vi "mfcc.vi"(1 "resoluci—n frec":dbl=21.533203125, 2 "PSD":dbl[](graph)=[3.9887404437067745e-08, 4.863361306709987e-06, 1.3039418095344414e-05, 5.070012021923156e-06, 2.6988740160259597e-08, 9.26549526636648e-08, 3.8708700843128457e-07, 5.27273770508995e-07, 1.8373351232795647e-07, 2.6971849055927445e-08, 1.1305706015574627e-07, 3.806307699408786e-08, 2.0069416323355392e-07, 2.823609797855514e-08, 5.568307171527192e-07, 4.654751624780882e-07, 1.8592522762634433e-07, 7.805098623746083e-09, 7.415656034335313e-08, 8.618601809462274e-08, 8.367973007840736e-09, 2.741395830035607e-09, 1.29708294460803e-08, 4.94468548724558e-08, 4.2508491067198684e-08, 2.5345057363752737e-09, 5.384088622693212e-09, 4.567329467519097e-10, 4.589634256892734e-08, 8.061224081254841e-08, 4.9934089467380857e-08, 4.900251155663863e-08, 6.064620630253797e-08, 1.3977491793314023e-08, 1.2377637981365425e-08, 1.2830909334877326e-08, 1.2367865096283767e-08, 2.2310979820652065e-09, 5.329299843141029e-10, 8.358860058537406e-10, 2.7965160679452414e-09, 8.57666812976728e-09, 5.0904982945537655e-09, 1.850249424215745e-08, 6.567181023968075e-09, 1.1774111924438839e-08, 2.5791701765030143e-08, 1.982423640874352e-08, 5.419962767506519e-09, 4.1419899242594406e-09, 4.689780545502817e-10, 6.653744223348867e-09, 2.6663411491893394e-08, 1.9381046099943884e-08, 3.4180900994948075e-09, 6.674963773837645e-09, 9.66181831593392e-09, 1.71947708792769e-08, 1.195261364973032e-08, 2.049897150446483e-09, 4.392273116033887e-10, 2.616427006264454e-09, 6.690001407319274e-09, 7.684978388820196e-09, 3.3903996771582425e-09, 1.2620299088279496e-09, 1.5781865769333585e-08, 6.835172346273258e-09, 4.279837116370928e-09, 1.017633364236646e-09, 1.5278934940047075e-09, 7.288208655911123e-10, 5.677716902112507e-10, 3.686854781768968e-10, 1.2948045853382716e-09, 6.441644862826187e-11, 1.7379620768753635e-09, 9.67268154903921e-08, 1.5926146703086817e-07, 1.84839387576239e-08, 1.5514964942226702e-10, 3.6806446299820845e-10, 6.391088644654868e-10, 1.2100481419233764e-09, 1.578433777229095e-09, 1.56615998978063e-09, 1.6356209328902429e-09, 7.968851827673522e-10, 1.048883110359278e-10, 3.154548207484171e-10, 6.72086666489939e-11, 5.562586170593403e-10, 1.7466042145935007e-10, 4.480068289721987e-10, 4.143358107708358e-10, 6.668260473459438e-11, 1.166302512750863e-10, 8.292201135724018e-10, 3.3781116752592635e-10, 1.388955298270216e-10, 4.1396624586413795e-10, 3.227466924577699e-10, 1.0493479042861911e-10, 1.1775778471972923e-10, 9.424146957824344e-11, 2.562400516107372e-13, 3.178514317358408e-11, 1.1402815490884768e-10, 2.593014170581146e-11, 1.0387827844257038e-10, 1.9555196850340233e-10, 9.399804236122056e-11, 1.8273331201730445e-11, 2.8943679934456845e-11, 1.2548464745442652e-10, 5.7404252467202236e-11, 3.583082697816324e-11, 1.0074456051377992e-10, 9.095619866099985e-11, 1.9214591454073945e-11, 1.7653596131622882e-11, 2.3767814754529185e-12, 2.6607109775921123e-11, 2.2175044068335442e-11, 1.1690124555337247e-11, 4.7761790450858616e-11, 4.152302479914363e-11, 5.744090546714635e-12, 6.4683935263009924e-12, 1.1770787831096862e-12, 4.5604502171813085e-12, 1.0081093160672481e-11, 2.613149358671662e-12, 1.3482181950104903e-11, 1.1131001635288938e-12, 2.5930316436774895e-11, 2.2617889198053044e-11, 3.0555023298879805e-11, 1.2999813512856096e-10, 1.1342969649559696e-10, 3.401389256701131e-11, 1.709914916053185e-11, 2.4422679377509385e-12, 1.6555985492742527e-12, 6.264935903608755e-12, 4.015636408815974e-12, 9.743669817695263e-12, 1.9242639981813654e-11, 9.976037495847763e-12, 1.065334544865495e-12, 7.606626156361599e-13, 4.924272167651513e-12, 2.7369335129743866e-12, 3.3145210049964618e-12, 8.612410770954802e-12, 3.0322149259003043e-11, 3.1739545043346e-11, 6.513310204922844e-12, 1.1414676387609523e-12, 2.531973410924266e-12, 1.4517312483736793e-12, 6.728687437136567e-13, 3.512934197758202e-12, 6.7694397609691784e-12, 2.5436294029964264e-12, 9.36548387216544e-14, 2.1181989376456617e-13, 2.7922718704211927e-12, 2.4572862907431585e-12, 6.358720838241306e-13, 1.096469033798667e-13, 8.04078486281365e-14, 6.568273396547891e-14, 3.0363326253607965e-13, 1.2274576171281992e-13, 2.620046007081006e-13, 7.151816142508422e-13, 6.602609191590688e-13, 3.699049093123982e-13, 2.67134170631445e-13, 1.9180325998924723e-13, 1.016892059083577e-12, 8.897650774215133e-13, 6.56588606025403e-13, 4.742616930979475e-13, 3.078597604428613e-13, 5.939345283269445e-13, 2.3000742821822784e-13, 1.4609087868974407e-14, 4.317013227907856e-13, 9.846963276825253e-14, 1.5677417688049744e-13, 3.9427819306671406e-13, 2.964979831861804e-13, 1.8693132619095558e-13, 6.028345235016743e-13, 1.531064938243066e-13, 4.760493615794276e-14, 5.107677831604972e-14, 7.00201959190453e-14, 1.1336557135022641e-13, 1.8416324608154718e-14, 1.901454612484762e-14, 9.175808956023227e-14, 2.995603678750294e-13, 3.9479268033615506e-13, 6.675790986865387e-14, 3.056239941978787e-13, 4.739145759584094e-13, 2.4519025793727183e-13, 3.4211508571711695e-13, 1.241858015730373e-13, 4.5106047230269066e-13, 1.809029526361038e-12, 2.1876693063718996e-12, 9.502314466220182e-13, 2.0019550009823214e-13, 7.654970848409915e-13, 5.634793901127196e-13, 3.6460638614428325e-14, 4.3896059912585293e-13, 9.34075341892215e-13, 2.8287552921420905e-13, 1.6831750650904512e-13, 5.375877985958264e-13, 5.447797492587748e-13, 1.0952620201643962e-13, 3.431962598080462e-14, 1.9476590484137924e-14, 1.9648081293354594e-13, 4.5363229271909907e-13, 7.781284392009688e-14, 3.1991422620776933e-15, 9.954971787069777e-13, 2.095751893127129e-12, 1.0162630181859588e-12, 1.486558214237754e-13, 1.7621053567422038e-13, 6.411969857406429e-13, 9.71443420295746e-13, 1.2182029481081724e-12, 8.727362158206555e-13, 2.7530277597716464e-13, 2.0337111581433584e-13, 7.595997700470152e-13, 4.147465407508831e-13, 1.0535136119615071e-12, 4.1053106258452134e-13, 8.505479272567457e-13, 7.072034534051268e-13, 9.772040146329993e-15, 6.351334119875336e-15, 2.001985367977675e-13, 5.645013333631312e-13, 3.724724445027121e-13, 5.955400706558533e-14, 4.572628365172749e-15, 2.996300881734785e-14, 3.7332143954694604e-14, 1.4097753371238528e-14, 8.19143375291366e-14, 4.783308863301145e-14, 3.992758327056385e-14, 4.766225492972332e-14, 7.957452766646809e-15, 3.0257523884900864e-14, 3.689177778626434e-15, 2.909528666318849e-14, 2.3280985274795645e-15, 8.671371216942672e-15, 2.048119252857748e-14, 2.0486343153893224e-14, 3.3908187771523714e-15, 6.816660644170723e-16, 1.2766402859232343e-14, 1.588251761923619e-15, 2.35734732041747e-15, 1.0750448782601794e-14, 1.4071103075169076e-14, 2.5669416702513182e-14, 1.1619006145640397e-15, 6.480493120678063e-14, 4.1535974359725746e-14, 4.0147122068886274e-14, 6.111486222691414e-14, 9.90541212064997e-14, 4.523302306273945e-14, 2.598729497645613e-14, 2.4781241053992947e-15, 1.924030634852899e-14, 3.186922326540168e-14, 2.0381706156419735e-14, 1.442941901249693e-14, 1.6951060118713328e-14, 2.8154409808082236e-14, 4.8874407961357667e-14, 4.0739817438194013e-14, 1.7398559081301259e-12, 3.1575096274050193e-12, 8.148821730169221e-13, 7.443600852166219e-14, 1.859865861756136e-14, 4.99842038203551e-16, 6.907476053584001e-14, 1.211080249932455e-13, 9.984491160248407e-14, 1.4752232424661912e-13, 4.596568054722706e-14, 6.134920453411187e-14, 9.803872952879367e-14, 2.3600314209981603e-13, 3.370049276879626e-13, 1.2813370676586174e-13, 9.810113817322674e-14, 8.530712737210603e-14, 4.161323330057365e-14, 6.544847509409676e-14, 4.1626336315984065e-14, 6.646410192084647e-14, 2.0633377435958723e-14, 3.472821009538355e-14, 3.94647958325078e-14, 2.474007622348129e-14, 8.8698028574754e-14, 1.5504681285081675e-14, 1.0469877253385006e-13, 7.81492504658662e-14, 1.2808778841569757e-13, 7.971741581476955e-14, 5.509197921916587e-14, 1.1215688354830048e-13, 3.383707123407506e-14, 1.6538965354317382e-15, 1.9656444729553843e-15, 1.663238725815441e-14, 5.454241212590961e-15, 3.655657840082562e-16, 2.78345472522134e-14, 7.167635432911245e-15, 3.325028129591217e-14, 7.613870201779507e-14, 7.246830754872868e-14, 9.84919690220968e-14, 2.918037144579805e-14, 1.0018003712149877e-13, 6.1121352397607724e-15, 1.7144544856159762e-15, 1.9862858918173206e-14, 2.451594976103451e-14, 1.2912658788526311e-14, 1.6989256578624025e-15, 4.816001466063061e-14, 4.338212442417716e-14, 7.710510986182302e-14, 4.138052677959718e-14, 7.233586630406715e-14, 3.606668524680535e-14, 1.3170176001518041e-15, 3.047221269426907e-15, 3.8039609228610015e-15, 1.197054977399816e-15, 1.622562201094902e-15, 1.2797534408003715e-14, 2.8561781073823506e-15, 1.5475472893006592e-14, 2.89110266752069e-14, 1.294182737098977e-14, 2.3043753883543014e-16, 9.108501275383515e-15, 4.785450146638445e-15, 2.7009905929641626e-14, 3.377919583930731e-14, 4.751948731293581e-14, 1.152394992558849e-13, 4.0750837788540076e-14, 5.3601526749334667e-14, 1.0736676012024376e-14, 1.6695853074324793e-16, 3.9071944414848e-17, 1.9285876705276466e-15, 1.5258612591104148e-14, 4.186564864740511e-14, 1.550013238457319e-14, 8.879820150711253e-15, 4.789920063096019e-15, 6.082358323961749e-14, 3.1937771920260896e-14, 4.274987996446661e-14, 2.998287958805335e-14, 6.995205996301659e-16, 1.6396121969311354e-14, 6.313846352858399e-15, 1.81502939655127e-15, 2.016365585590927e-16, 1.984961509651681e-15, 5.588569581038433e-15, 2.0078800032452958e-16, 1.7399294929161574e-15, 2.823509550449133e-15, 1.4349215246825145e-14, 8.413146789264872e-15, 6.997529352579209e-15, 9.218777520117128e-15, 3.131725123349588e-15, 1.3484862021439288e-14, 2.3516394321778644e-14, 5.526764756732445e-14, 6.7159669069588e-14, 3.176557762522999e-14, 1.0401787524399212e-13, 6.262074247012217e-14, 1.815537153265782e-14, 1.8872886243220736e-15, 6.30856774949859e-15, 7.452086950198022e-15, 9.092019303237341e-14, 6.452652978689391e-14, 1.0518011621021188e-13, 1.45807147724322e-13, 1.3824596740645433e-13, 1.8219055585463523e-13, 1.1252613268664737e-13, 9.43946580874044e-14, 1.3730365294555875e-13, 5.761515967539565e-14, 2.002631162872167e-14, 7.223657431422928e-15, 1.2176496682290998e-16, 6.975640035821606e-15, 1.6633740056757412e-14, 2.53300200333288e-15, 1.8380633604829153e-15, 1.948603850345286e-14, 4.246779951276348e-15, 2.3498357836878853e-14, 5.4730819770021296e-15, 2.7627825870497137e-14, 5.0904577157370106e-15, 1.7244435435100095e-14, 6.226678240490165e-15, 7.330217162306043e-15, 3.2391405728917565e-15, 6.944508501967592e-15, 2.08927506067488e-14, 1.85672034522362e-14, 6.737610874913574e-14, 8.517628550511586e-14, 6.767306215637752e-14, 2.6665614045781447e-14, 2.1771261642041072e-14, 2.1079997606339945e-15, 5.778199455299098e-15, 2.0474480581576226e-15, 1.1014388535233335e-14, 2.8585792141883013e-15, 3.9429940450870805e-16, 2.112665458806322e-15, 7.84600165059488e-15, 6.992386028372992e-16, 3.593228350282517e-15, 8.375674606135625e-16, 6.0091781824076144e-15, 3.4119153483839917e-15, 1.6616143603589067e-14, 4.3110032816606783e-14, 4.7608178196160537e-14, 4.170937761544873e-14, 3.965989713889973e-14, 3.9441900318178696e-14, 2.1667086740329935e-14, 9.20978912637376e-16, 5.591043378196642e-15, 1.430533914811028e-14, 1.955611421106458e-14, 1.9661283688968425e-15, 2.7313487489613825e-15, 7.218988204632122e-15, 1.2066707606118975e-15, 1.7822150935267495e-14, 3.061025540844946e-14, 2.601589381267546e-15, 3.36846779350327e-14, 5.464786373112407e-15, 4.919076333263889e-14, 6.991083244976793e-14, 1.282693148967392e-13, 9.763113482307137e-14, 1.170096944471583e-13, 4.207201595636027e-14, 2.5318020579554097e-14, 9.045085913796983e-15, 8.478928177238485e-15, 1.6210453572276712e-14, 2.5313143665707674e-14, 5.0406048271773305e-14, 1.2473292584210862e-14, 6.0847598279728585e-15, 1.6739087139713107e-14, 3.0564069131820365e-14, 2.2397581743816812e-15, 7.827296264383575e-14, 1.3600511565900048e-14, 5.6218567267975764e-14, 8.005380453623486e-14, 2.7785501166962964e-15, 1.4992922529608968e-14, 1.2865291229366007e-14, 6.233603641875634e-15, 2.4208643099664175e-15, 1.872798250536615e-14, 2.1982196700892394e-14, 3.476642338057269e-14, 6.434674416000958e-14, 5.1227126819268735e-14, 7.207533817451576e-14, 5.063626409437162e-14, 4.8381793294746975e-14, 2.440228060570871e-14, 8.711029313737643e-15, 4.825231975894077e-14, 5.1505514148909e-14, 5.461763707899197e-15, 2.7427477857547005e-14, 4.477275117760359e-15, 4.109748958060314e-15, 9.54157692354231e-16, 2.0464198638754147e-15, 2.1879750629295906e-15, 1.0961111872738179e-14, 7.067854269043573e-15, 2.5621428575758327e-14, 1.2891768885721538e-14, 2.9022952717105004e-15, 7.085304315919362e-16, 5.52052851992987e-15, 1.0635180977139302e-14, 9.312451292053164e-15, 8.954848417652913e-15, 1.211591792654409e-15, 7.437026757498448e-15, 1.851731562339207e-14, 6.556339551298976e-15, 2.0261193319341016e-15, 6.990073186467462e-15, 3.366949637544587e-15, 1.185496653386074e-15, 1.0180667665884057e-15, 4.7336660656794555e-15, 7.367309744337908e-15, 1.0093467140054865e-15, 3.2124788682320108e-15, 2.7659266271876152e-15, 2.1481838557236626e-15, 5.5547367065160524e-15, 7.477340516013398e-16, 6.471232351725521e-15, 4.335615564722991e-15, 5.259738697830469e-15, 2.4946023544002045e-15, 2.150900532546934e-15, 4.038516744060081e-15, 6.924350098827874e-15, 5.051521386071476e-15, 3.661773430359469e-15, 2.2580348216753544e-15, 6.550386916045646e-15, 1.0009597014894823e-14, 6.4523787900459176e-15, 4.227183659921416e-15, 3.2430485208371364e-15, 4.1751316707034456e-15, 8.878358065239006e-16, 2.959751900890256e-15, 5.20520294376908e-15, 1.2393932768829355e-15, 4.3970148439658814e-15, 8.320329007426342e-15, 8.865432991446226e-15, 5.983343315141536e-15, 7.477513516625403e-15, 4.611589794997294e-15, 8.623545579570438e-16, 7.454461716882186e-16, 7.295961627816521e-16, 9.671450506643574e-16, 9.987482396233898e-15, 1.9958724021488275e-14, 1.8459173323289555e-15, 6.406803970801615e-15, 1.554568451113529e-14, 8.13499560187335e-15, 2.743710424280864e-15, 2.6684750426379986e-15, 1.0107128185160135e-15, 8.114024432167224e-15, 3.2935898985201707e-15, 1.8708944702423912e-15, 3.9882321960437e-15, 1.3311731003442253e-15, 1.7541289016104554e-15, 2.0329393364231603e-15, 8.383508347526691e-16, 2.298827376287461e-15, 2.8172844215643272e-15, 5.338352833510282e-15, 2.1340230335894928e-15, 2.285102688433937e-15, 3.684538382467707e-15, 1.3151534438644683e-15, 1.0543194328283072e-16, 1.6138895638921527e-15, 3.551993260265015e-15, 1.8599150456458737e-15, 4.1167034599470384e-15]) -> (0 "mezcla":dbl[](graph))   [LabVIEW 2010]
uses:
  <vilib>/Analysis/2dsp.llb/1D DCT.vi
  <vilib>/Analysis/NI_AALPro.lvlib
panel:
  in  "n coefs salida":dbl=20.0
  in  "N filtros log":dbl=30.0
  in  "N filtros lineal":dbl=18.0
  in  "Incremento ancho banda log":dbl=1.107
  in  "Ancho de banda lineal":dbl=63.0
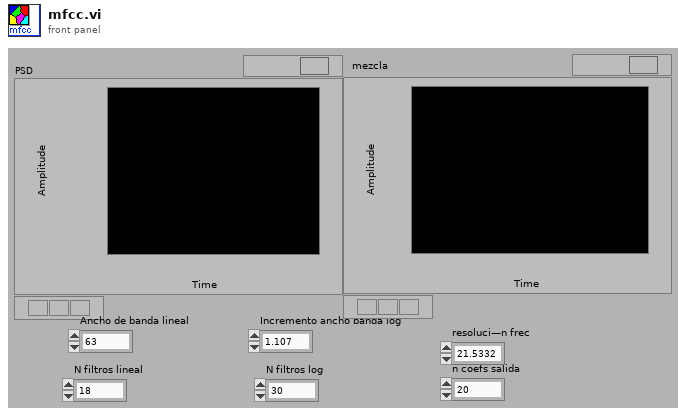
[diagram p1: front panel]
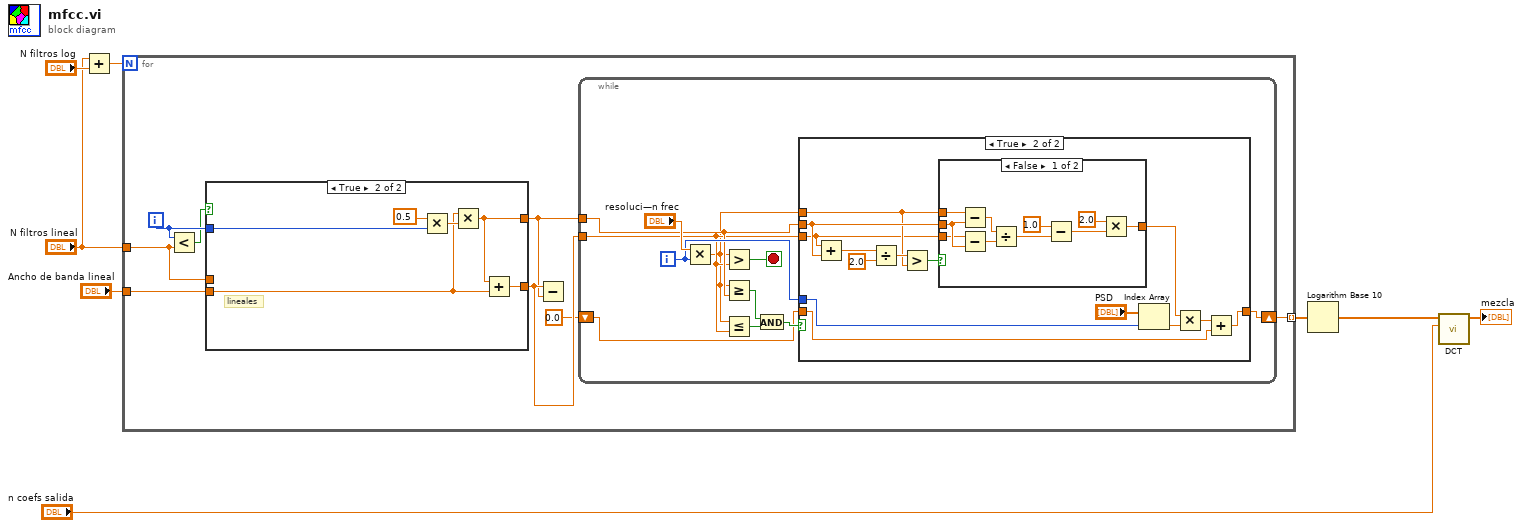
[diagram p0: block diagram]
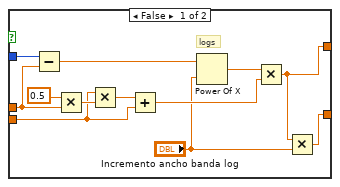
[diagram p2: hidden frame]
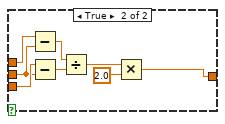
[diagram p4: hidden frame]
diagram:
  n1 = Add(x="N filtros lineal", y="N filtros log") -> (x+y=w8:dbl)
  n2 = for {
    N: w8 -> [_]
    tunnel: [w9] -> w3 mode=indexing
    tunnel: "N filtros lineal" -> [w14]
    tunnel: "Ancho de banda lineal" -> [w15]
    i -> [w16]
    n3 = Less?(x=w16, y=w14) -> (x < y?=w13:bool)
    n4 = case shown="True" w13 {
      tunnel: w16 -> [w24 w34]
      tunnel: [w19 w31] -> w11
      tunnel: [w17 w30] -> w12
      tunnel: w15 -> [w25 w29]
      tunnel: w14 -> [w23 _]
      frame False {
        # "logs"
        n5 = Subtract(x=w24, y=w23) -> (x-y=w22:dbl)
        n6 = Multiply(x=0.5, y=w23) -> (x*y=w28:dbl)
        n7 = Multiply(x=w25, y=w28) -> (x*y=w26:dbl)
        n8 = Add(x=w26, y=w25) -> (x+y=w20:dbl)
        n9 = Power Of X(1:"Incremento ancho banda log", 2:w22) -> (0:w21:dbl)
        n10 = Multiply(x=w21, y=w20) -> (x*y=w19:dbl)
        n11 = Multiply(x=w19, y="Incremento ancho banda log") -> (x*y=w17:dbl)
      }
      frame True {
        # "lineales"
        n12 = Multiply(x=0.5, y=w34) -> (x*y=w33:dbl)
        n13 = Multiply(x=w29, y=w33) -> (x*y=w31:dbl)
        n14 = Add(x=w31, y=w29) -> (x+y=w30:dbl)
      }
    }
    n15 = Subtract(x=w12, y=w11) -> ()  [unwired: 1 out]
    n16 = while {
      tunnel: w11 -> [w37]
      tunnel: w12 -> [w36]
      shift-right: [w39] -> w9
      shift-left: 0.0 -> [w38]
      i -> [w40]
      stop <- w44 stop-if-true
      n17 = Multiply(x="resoluci—n frec", y=w40) -> (x*y=w35:dbl)
      n18 = Greater?(x=w35, y=w36) -> (0:w44:bool)
      n19 = Greater Or Equal?(x=w35, y=w37) -> (x >= y?=w42:bool)
      n20 = Less Or Equal?(x=w35, y=w36) -> (x <= y?=w41:bool)
      n21 = And(x=w42, y=w41) -> (x .and. y?=w43:bool)
      n22 = case shown="True" w43 {
        tunnel: w40 -> [_ w60]
        tunnel: [w46 w59] -> w39
        tunnel: w38 -> [w46 w58]
        tunnel: w37 -> [_ w52]
        tunnel: w36 -> [_ w50]
        tunnel: w35 -> [_ w51]
        frame False {
        }
        frame True {
          n23 = Add(x=w50, y=w52) -> (x+y=w56:dbl)
          n24 = Divide(x=w56, y=2.0) -> (x/y=w54:dbl)
          n25 = Greater?(x=w54, y=w51) -> (0:w53:bool)
          n26 = case shown="False" w53 {
            tunnel: w52 -> [w67 w76]
            tunnel: w51 -> [w68 w78]
            tunnel: w50 -> [w66 w77]
            tunnel: [w61 w72] -> w48
            frame False {
              n27 = Subtract(x=w68, y=w67) -> (x-y=w69:dbl)
              n28 = Subtract(x=w66, y=w67) -> (x-y=w70:dbl)
              n29 = Divide(x=w69, y=w70) -> (x/y=w64:dbl)
              n30 = Subtract(x=1.0, y=w64) -> (x-y=w63:dbl)
              n31 = Multiply(x=2.0, y=w63) -> (x*y=w61:dbl)
            }
            frame True {
              n32 = Subtract(x=w78, y=w76) -> (x-y=w74:dbl)
              n33 = Subtract(x=w77, y=w76) -> (x-y=w75:dbl)
              n34 = Divide(x=w74, y=w75) -> (x/y=w73:dbl)
              n35 = Multiply(x=w73, y=2.0) -> (x*y=w72:dbl)
            }
          }
          n36 = Index Array(array="PSD", index=w60) -> (element=w49:dbl)
          n37 = Multiply(x=w48, y=w49) -> (x*y=w47:dbl)
          n38 = Add(x=w47, y=w58) -> (x+y=w59:dbl)
        }
      }
    }
  }
  n39 = Logarithm Base 10(1:w3) -> (0:w2:dbl[])
  n40 = call-poly <vilib>:"DCT.vi"("DCT size"="n coefs salida", "X"=w2) -> ("DCT {X}"=→"mezcla":dbl[])  [unwired: 8 in, 1 out]
